vi "Test Save TGA (Path).vi"(8 "error in (no error)":errorcluster) -> (0 "error out":errorcluster, 3 "Pass?":bool)   [LabVIEW 2020]
uses:
  <vilib>/picture/picture.llb/imagedata.ctl
  G-Image/Image IO/Polymorphic VIs/Load Image (Path).vi
  G-Image/G-Image.lvlib
  G-Image/Image IO/Polymorphic VIs/Save TGA Image (Path).vi
panel:
  out "Array":cluster{string, "new picture":picture}[](array[cluster])
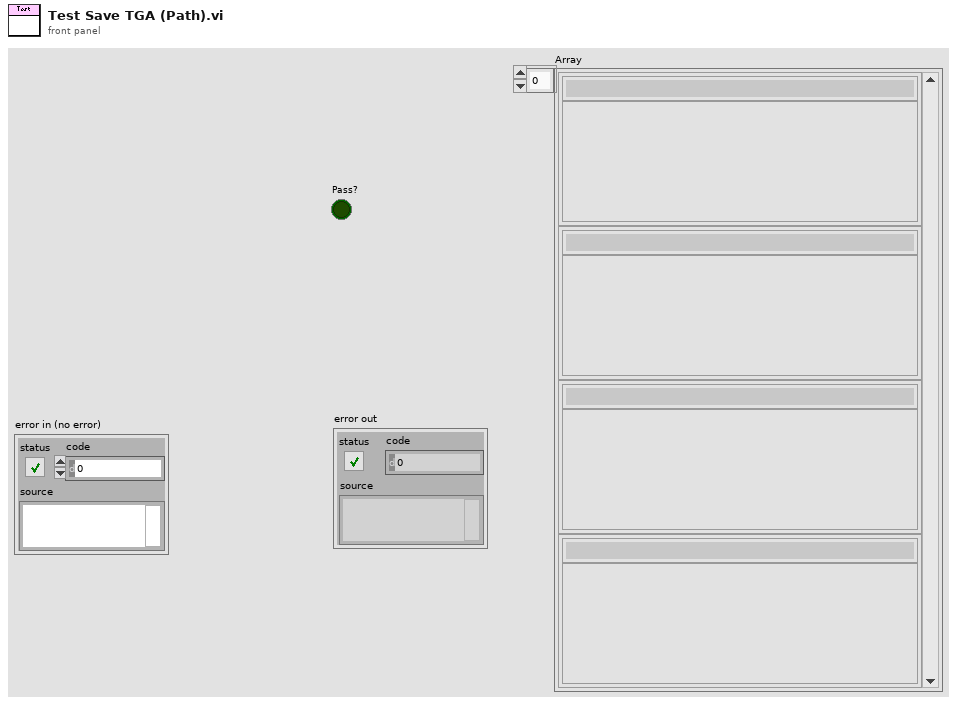
[diagram p1: front panel]
types:
  T1 = typedef "imagedata.ctl" = cluster{"image type":i32, "image depth":i32, "image":u8[], "mask":u8[], "colors":u32[], "Rectangle":cluster{"left":i16, "top":i16, "right":i16, "bottom":i16}}
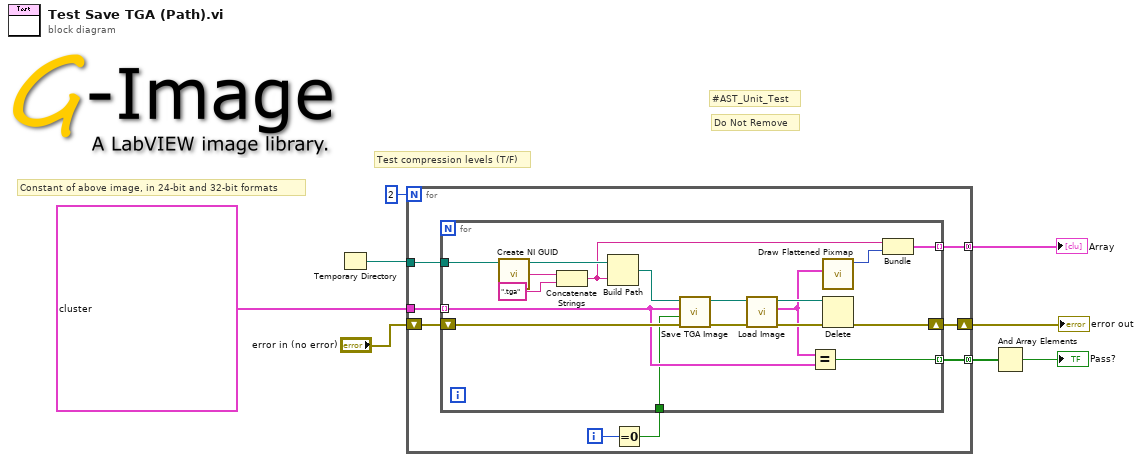
[diagram p0: block diagram]
diagram:
  # "Test compression levels (T/F)"
  # "Constant of above image, in 24-bit and 32-bit formats"
  # "Do Not Remove"
  # "#AST_Unit_Test"
  n1 = Temporary Directory() -> (w7:path)
  n2 = for {
    N: 2 -> [_]
    tunnel: w7 -> [w15]
    tunnel: [w14] -> w6 mode=concatenating
    tunnel: [w12] -> w4 mode=concatenating
    tunnel: T1[] [{"image type"=0, "image depth"=24, "image"=array[115500 elements], "mask"=[], "colors"=[], "Rectangle"={"left"=0, "top"=0, "right"=350, "bottom"=110}}, {"image type"=0, "image depth"=32, "image"=array[154000 elements], "mask"=array[4840 elements], "colors"=[], "Rectangle"={"left"=0, "top"=0, "right"=350, "bottom"=110}}] ("Array 2") -> [w11]
    shift-right: [w13] -> w5
    shift-left: "error in (no error)" -> [w16]
    i -> [w10]
    n3 = Equal To 0?(x=w10) -> (x = 0?=w9:bool)
    n4 = for {
      tunnel: w15 -> [w30]
      tunnel: w11 -> [w26] mode=indexing
      shift-right: [w23] -> w13
      shift-left: w16 -> [w33]
      tunnel: [w22] -> w12 mode=indexing
      tunnel: [w18] -> w14 mode=indexing
      tunnel: w9 -> [w17]
      n5 = call <vilib>:"Create NI GUID.vi"() -> ("NI GUID"=w31:string)
      n6 = Concatenate Strings(w31, ".tga" ("string")) -> (w19:string)
      n7 = Build Path(base path=w30, name or relative path=w19) -> (appended path=w29:path)
      n8 = call-poly "Save TGA Image.vi"("error in (no error)"=w33, "Compress (T)"=w17, "Image"=w26, "Path In"=w29) -> ("error out"=w27:errorcluster, "Path Out"=w28:path)  [unwired: 6 in]
      n9 = call-poly "Load Image.vi"("error in (no error)"=w27, "Path In"=w28) -> ("error out"=w24:errorcluster, "Image"=w21:T1, "Path Out"=w25:path)  [unwired: 7 in]
      n10 = Equal?(x=w21, y=w26) -> (x = y?=w22:bool)
      n11 = call <vilib>:"Draw Flattened Pixmap.vi"("image data"=w21) -> ("new picture"=w20:picture)  [unwired: 8 in]
      n12 = Delete(path (use dialog)=w25, error in=w24) -> (error out=w23:errorcluster)  [unwired: 3 in, 2 out]
      n13 = Bundle(w19, "new picture"=w20) -> (w18:cluster{string, "new picture":picture})  [unwired: 1 in]
    }
  }
  "error out" <- w5
  "Array" <- w6
  n14 = And Array Elements(Boolean array=w4) -> (logical AND=→"Pass?":bool)
